vi "PADMINI_varient_to_data.vi"(8 "error in (no error)":errorcluster, 11 "data":variant[][](array[variant])) -> (0 "error out":errorcluster, 3 "Array":string[][](array[string]))   [LabVIEW 2017]
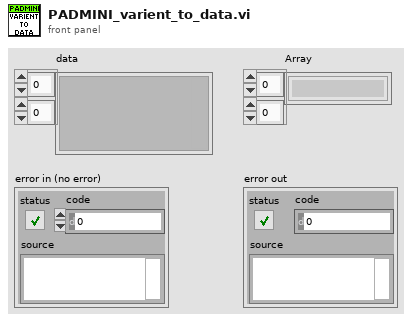
[diagram p1: front panel]
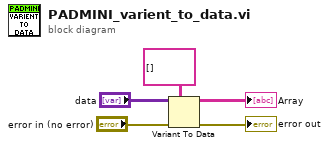
[diagram p0: block diagram]
diagram:
  n1 = Variant To Data(error in="error in (no error)", type=string[][] [], Variant="data") -> (data=→"Array":string[][], error out=→"error out":errorcluster)
